vi "PV ActiveLine - FilterTime (TPG361).vi"(7 "W/R":bool, 8 "Fehler (Eingang)":errorcluster, 10 "Sensor 1 Set":i8(ring)=2 items=["Filter off", "Fast", "Normal", "Slow"], 11 "Referenz in":refnum<visa-resource-name>) -> (0 "Cluster (Ausgang)":errorcluster, 2 "Sensor 1 Get":i8(ring)=2 items=["Filter off", "fast", "normal", "slow"], 3 "Referenz out":refnum<visa-resource-name>)   [LabVIEW 2013, in "PV ActiveLine.lvlib"]
doc: "FIL - Measurement Value Filter\n\nTransmit: FIL [,a]\nReceive: a\n\nFilter gauge 1,\na =\n0 –> Filter off\n1 –> Fast\n2 –> Normal\n3 –> Slow"
uses:
  C:/Program Files (x86)/National Instruments/LabVIEW 2013/PV ActiveLine/PV ActiveLine.lvlib
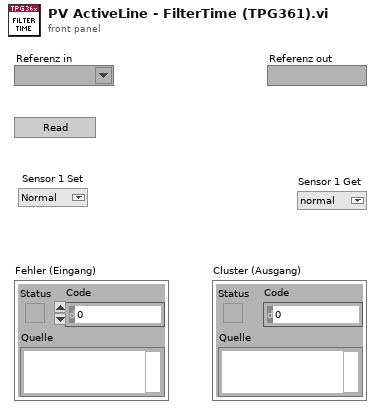
[diagram p1: front panel]
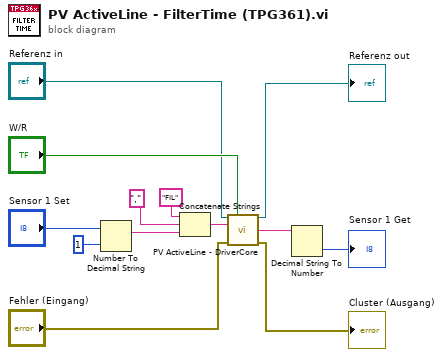
[diagram p0: block diagram]
diagram:
  n1 = Number To Decimal String(number="Sensor 1 Set", width (-)=i16 1) -> (decimal integer string=w3:string)
  n2 = Concatenate Strings("FIL", ",", w3) -> (w11:string)
  n3 = call "PV ActiveLine - DriverCore.vi"("Referenz in"="Referenz in", "Write/Read"="W/R", "Command"=w11, "Fehler (Eingang)"="Fehler (Eingang)") -> ("Referenz out"=→"Referenz out":refnum<visa-resource-name>, "String Out"=w2:string, "Cluster (Ausgang)"=→"Cluster (Ausgang)":errorcluster)  [unwired: 9 in]
  n4 = Decimal String To Number(string=w2) -> (number=→"Sensor 1 Get":i32)  [unwired: 2 in, 1 out]
